vi "FRIC_navX_Get_RawValues_GyroAccelMag.vi"(5 "Device Number":T1, 7 "Update":bool) -> (2 "Raw Values (out)":T2)   [LabVIEW 2016]
doc: "This navX VI returns the raw values from the Gyro, Accel, and Mag sensors."
uses:
  _TypeDefs/FRIC_navX_DeviceNumbersTypeDef.ctl
  _TypeDefs/Z900_navX_DeviceRegisters.ctl
  _Util/Z900_navX_Util_LittleEndian_to_BigEndian.vi
  _Internal/FRIC_navX_Get_Registry.vi
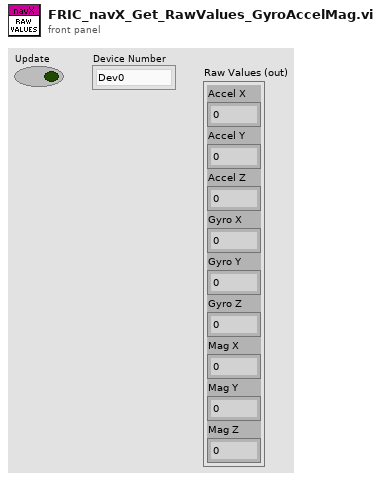
[diagram p1: front panel]
types:
  T1 = typedef "FRIC_navX_DeviceNumbersTypeDef.ctl" = enum16{"Dev0", "Dev1", "Dev2", "Dev3"}
  T2 = cluster{"Accel X":dbl, "Accel Y":dbl, "Accel Z":dbl, "Gyro X":dbl, "Gyro Y":dbl, "Gyro Z":dbl, "Mag X":dbl, "Mag Y":dbl, "Mag Z":dbl}
  T3 = typedef "Z900_navX_DeviceRegisters.ctl" = u8
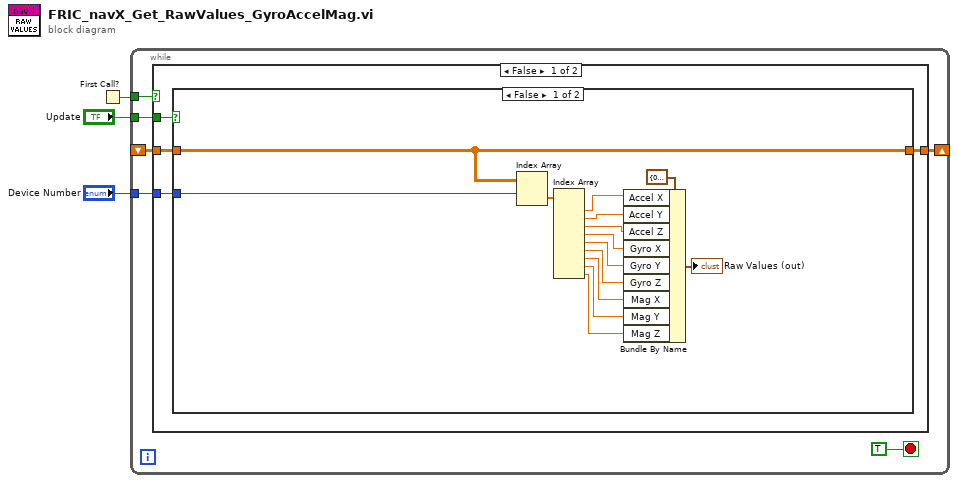
[diagram p0: block diagram]
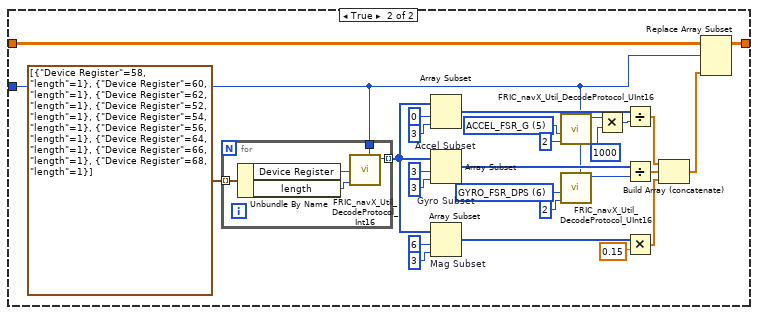
[diagram p2: hidden frame]
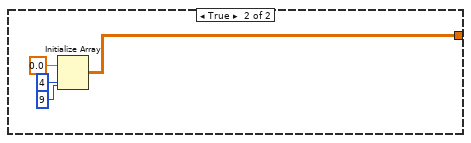
[diagram p3: hidden frame]
diagram:
  n1 = First Call?() -> (First Call?: T/F=w2:bool)
  n2 = while {
    shift-right: [w9] -> _
    shift-left: _ -> [w6]
    tunnel: "Update" -> [w7]
    tunnel: "Device Number" -> [w5]
    tunnel: w2 -> [w4]
    stop <- TRUE stop-if-true
    n3 = case shown="False" w4 {
      tunnel: [w13 w62] -> w9
      tunnel: w7 -> [w12 _]
      tunnel: w6 -> [w11 _]
      tunnel: w5 -> [w10 _]
      frame False {
        n4 = case shown="False" w12 {
          tunnel: [w15 w30] -> w13
          tunnel: w11 -> [w15 w31]
          tunnel: w10 -> [w14 w29]
          frame False {
            n5 = Index Array(array=w15, index (row)=w14) -> (element=w16:dbl[])  [unwired: 1 in]
            n6 = Index Array(array=w16) -> (element #1=w18:dbl, element #2=w19:dbl, element #3=w20:dbl, element #4=w21:dbl, element #5=w22:dbl, element #6=w23:dbl, element #7=w24:dbl, element #8=w25:dbl, element #9=w26:dbl)  [unwired: 9 in]
            n7 = Bundle By Name(cluster=T2 {"Accel X"=0.0, "Accel Y"=0.0, "Accel Z"=0.0, "Gyro X"=0.0, "Gyro Y"=0.0, "Gyro Z"=0.0, "Mag X"=0.0, "Mag Y"=0.0, "Mag Z"=0.0}, "Accel X"=w18, "Accel Y"=w19, "Accel Z"=w20, "Gyro X"=w21, "Gyro Y"=w22, "Gyro Z"=w23, "Mag X"=w24, "Mag Y"=w25, "Mag Z"=w26) -> (→"Raw Values (out)":T2)
          }
          frame True {
            w35 = T3 5 items=["WHOAMI"=0, "HW_REV"=1, "FW_VER_MAJOR"=2, "FW_VER_MINOR"=3, "UPDATE_RATE_HZ"=4, "ACCEL_FSR_G"=5, "GYRO_FSR_DPS"=6, "OP_STATUS"=8, "CAL_STATUS"=9, "SELFTEST_STATUS"=10, "CAPABILITY_FLAGS_L"=11, "CAPABILITY_FLAGS_H"=12, "SENSOR_STATUS"=16, "TIMESTAMP"=18, "YAW"=22, "ROLL"=24, "PITCH"=26, "HEADING"=28, "FUSED_HEADING"=30, "ALTITUDE_I"=32, "ALTITUDE_D"=34, "LINERA_ACC_X"=36, "LINERA_ACC_Y"=38, "LINERA_ACC_Z"=40, "QUAT_W"=42, "QUAT_X"=44, "QUAT_Y"=46, "QUAT_Z"=48, "MPU_TEMP_C"=50, "GYRO_X"=52, "GYRO_Y"=54, "GYRO_Z"=56, "ACC_X"=58, "ACC_Y"=60, "ACC_Z"=62, "MAG_X"=64, "MAG_Y"=66, "MAG_Z"=68, "PRESSURE_I"=70, "PRESSURE_D"=72, "PRESSURE_TEMP"=74, "YAW_OFFSET"=76, "QUAT_OFFSET_W"=78, "QUAT_OFFSET_X"=80, "QUAT_OFFSET_Y"=82, "QUAT_OFFSET_Z"=84, "INTEGRATION_CONTROL"=86, "VELOCITY_X"=88, "VELOCITY_Y"=92, "VELOCITY_Z"=96, "DISPLACMENT_X"=100, "DISPLACMENT_Y"=104, "DISPLACEMENT_Z"=108] ("Device Register")
            w39 = T3 6 items=["WHOAMI"=0, "HW_REV"=1, "FW_VER_MAJOR"=2, "FW_VER_MINOR"=3, "UPDATE_RATE_HZ"=4, "ACCEL_FSR_G"=5, "GYRO_FSR_DPS"=6, "OP_STATUS"=8, "CAL_STATUS"=9, "SELFTEST_STATUS"=10, "CAPABILITY_FLAGS_L"=11, "CAPABILITY_FLAGS_H"=12, "SENSOR_STATUS"=16, "TIMESTAMP"=18, "YAW"=22, "ROLL"=24, "PITCH"=26, "HEADING"=28, "FUSED_HEADING"=30, "ALTITUDE_I"=32, "ALTITUDE_D"=34, "LINERA_ACC_X"=36, "LINERA_ACC_Y"=38, "LINERA_ACC_Z"=40, "QUAT_W"=42, "QUAT_X"=44, "QUAT_Y"=46, "QUAT_Z"=48, "MPU_TEMP_C"=50, "GYRO_X"=52, "GYRO_Y"=54, "GYRO_Z"=56, "ACC_X"=58, "ACC_Y"=60, "ACC_Z"=62, "MAG_X"=64, "MAG_Y"=66, "MAG_Z"=68, "PRESSURE_I"=70, "PRESSURE_D"=72, "PRESSURE_TEMP"=74, "YAW_OFFSET"=76, "QUAT_OFFSET_W"=78, "QUAT_OFFSET_X"=80, "QUAT_OFFSET_Y"=82, "QUAT_OFFSET_Z"=84, "INTEGRATION_CONTROL"=86, "VELOCITY_X"=88, "VELOCITY_Y"=92, "VELOCITY_Z"=96, "DISPLACMENT_X"=100, "DISPLACMENT_Y"=104, "DISPLACEMENT_Z"=108] ("Device Register")
            n8 = for {
              tunnel: cluster{"Device Register":T3, "length":i32}[] [{"Device Register"=58, "length"=1}, {"Device Register"=60, "length"=1}, {"Device Register"=62, "length"=1}, {"Device Register"=52, "length"=1}, {"Device Register"=54, "length"=1}, {"Device Register"=56, "length"=1}, {"Device Register"=64, "length"=1}, {"Device Register"=66, "length"=1}, {"Device Register"=68, "length"=1}] ("Array") -> [w57] mode=indexing
              tunnel: [w56] -> w32 mode=indexing
              tunnel: w29 -> [w55]
              n9 = Unbundle By Name(w57) -> ("Device Register"=w59:T3, "length"=w58:i32)
              n10 = call "FRIC_navX_Util_DecodeProtocol_Int16.vi"("Device Number"=w55, "length"=w58, "Device Register"=w59) -> ("Value"=w56:i16)  [unwired: 8 in]
            }
            n11 = Array Subset "Accel Subset"(array=w32, index=0, length=3) -> (w48:i16[])
            n12 = Array Subset "Gyro Subset"(array=w32, index=3, length=3) -> (w47:i16[])
            n13 = Array Subset "Mag Subset"(array=w32, index=6, length=3) -> (w45:i16[])
            n14 = call "FRIC_navX_Util_DecodeProtocol_UInt16.vi"("Device Number"=w29, "length"=2, "Device Register"=w35) -> ("Value"=w33:u16)  [unwired: 8 in]
            n15 = call "FRIC_navX_Util_DecodeProtocol_UInt16.vi"("Device Number"=w29, "length"=2, "Device Register"=w39) -> ("Value"=w37:u16)  [unwired: 8 in]
            n16 = Multiply(x=w33, y=u16 1000) -> (x*y=w40:u16)
            n17 = Divide(x=w48, y=w40) -> (x/y=w44:dbl[])
            n18 = Divide(x=w47, y=w37) -> (x/y=w43:dbl[])
            n19 = Multiply(x=w45, y=0.15) -> (x*y=w42:dbl[])
            n20 = Build Array (concatenate)(w44, w43, w42) -> (w28:dbl[])
            n21 = Replace Array Subset(array=w31, new element=w28, index (row)=w29) -> (w30:dbl[][])  [unwired: 1 in]
          }
        }
      }
      frame True {
        n22 = Initialize Array(0.0, 4 ("dimension size"), 9 ("dimension size")) -> (w62:dbl[][])
      }
    }
  }
